vi "D020L_Motors.vi"() -> ()   [LabVIEW 2011]
uses:
  PIMotorController.llb/PI_Axis.ctl
panel:
  in  "PI Axis info":T2={"Piezo X"={"System #"=0, "Axis ID"=""}, "Piezo Y"={"System #"=0, "Axis ID"=""}, "Piezo Z"={"System #"=0, "Axis ID"="0"}, "Magnet Z"={"System #"=0, "Axis ID"="0"}, "Magnet Rotation"={"System #"=0, "Axis ID"="0"}, "Objective X"={"System #"=0, "Axis ID"=""}, "Objective Y"={"System #"=0, "Axis ID"=""}}
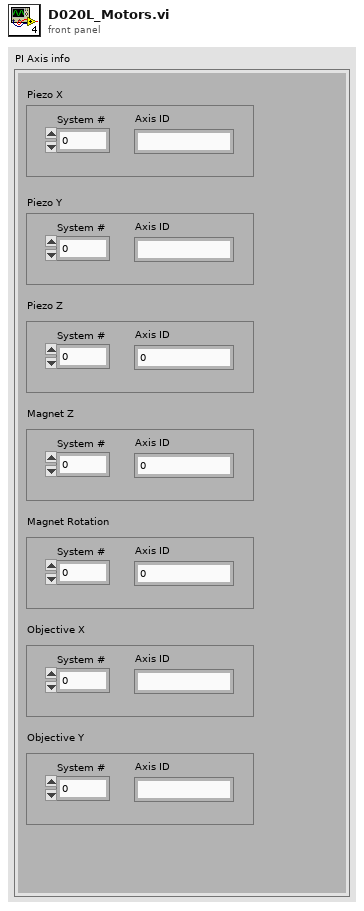
[diagram p1: front panel]
types:
  T1 = typedef "PI_Axis.ctl" = cluster{"System #":i32, "Axis ID":string}
  T2 = cluster{"Piezo X":T1, "Piezo Y":T1, "Piezo Z":T1, "Magnet Z":T1, "Magnet Rotation":T1, "Objective X":T1, "Objective Y":T1}
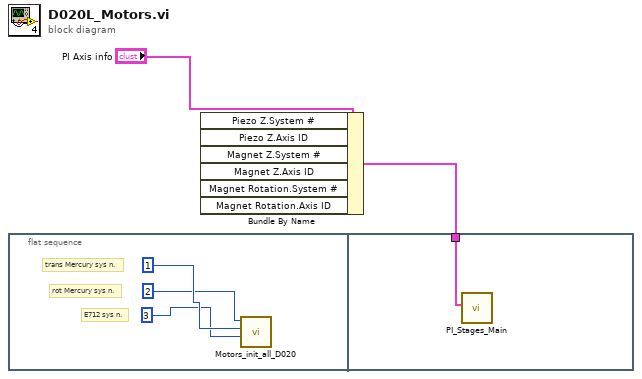
[diagram p0: block diagram]
diagram:
  n1 = flat-sequence {
    tunnel: w1 -> [w6]
    frame #0 {
      # "trans Mercury sys n."
      # "E712 sys n."
      # "rot Mercury sys n."
      n2 = call "Motors_init_all_D020.vi"("Mercury Rotation"=2 ("Mercury System no."), "Mercury Translation"=1 ("Mercury System no."), "E712 System no."=3) -> ()  [unwired: 2 in, 2 out]
    }
    frame #1 {
      n3 = call "PI_Stages_Main.vi"("PI Axis info"=w6) -> ()  [unwired: 11 in]
    }
  }
  n4 = Bundle By Name(cluster="PI Axis info") -> (w1:T2)  [unwired: 6 in]
